vi "Graph Display.vi"(10 "telem notifier":refnum<notifier>) -> ()   [LabVIEW 2015]
uses:
  Telemetry Packet Type.ctl
  Thermocouple Data.ctl
  Transducer Calibration Display.ctl
  Sensor Enum.ctl
  Sensor Data Global Action.ctl
panel:
  out "Timestamp":u32
  out "Air Pressure":dbl(graph)
  out "Compressor Temperature":dbl(graph)
  out "Article Temperature":dbl(graph)
  out "Accumulator Pressures":cluster{"FPD-2":dbl, "OPD-2":dbl}(graph)
  out "Chamber Pressure":cluster{"PC-2":dbl, "PC-1":dbl}(graph)
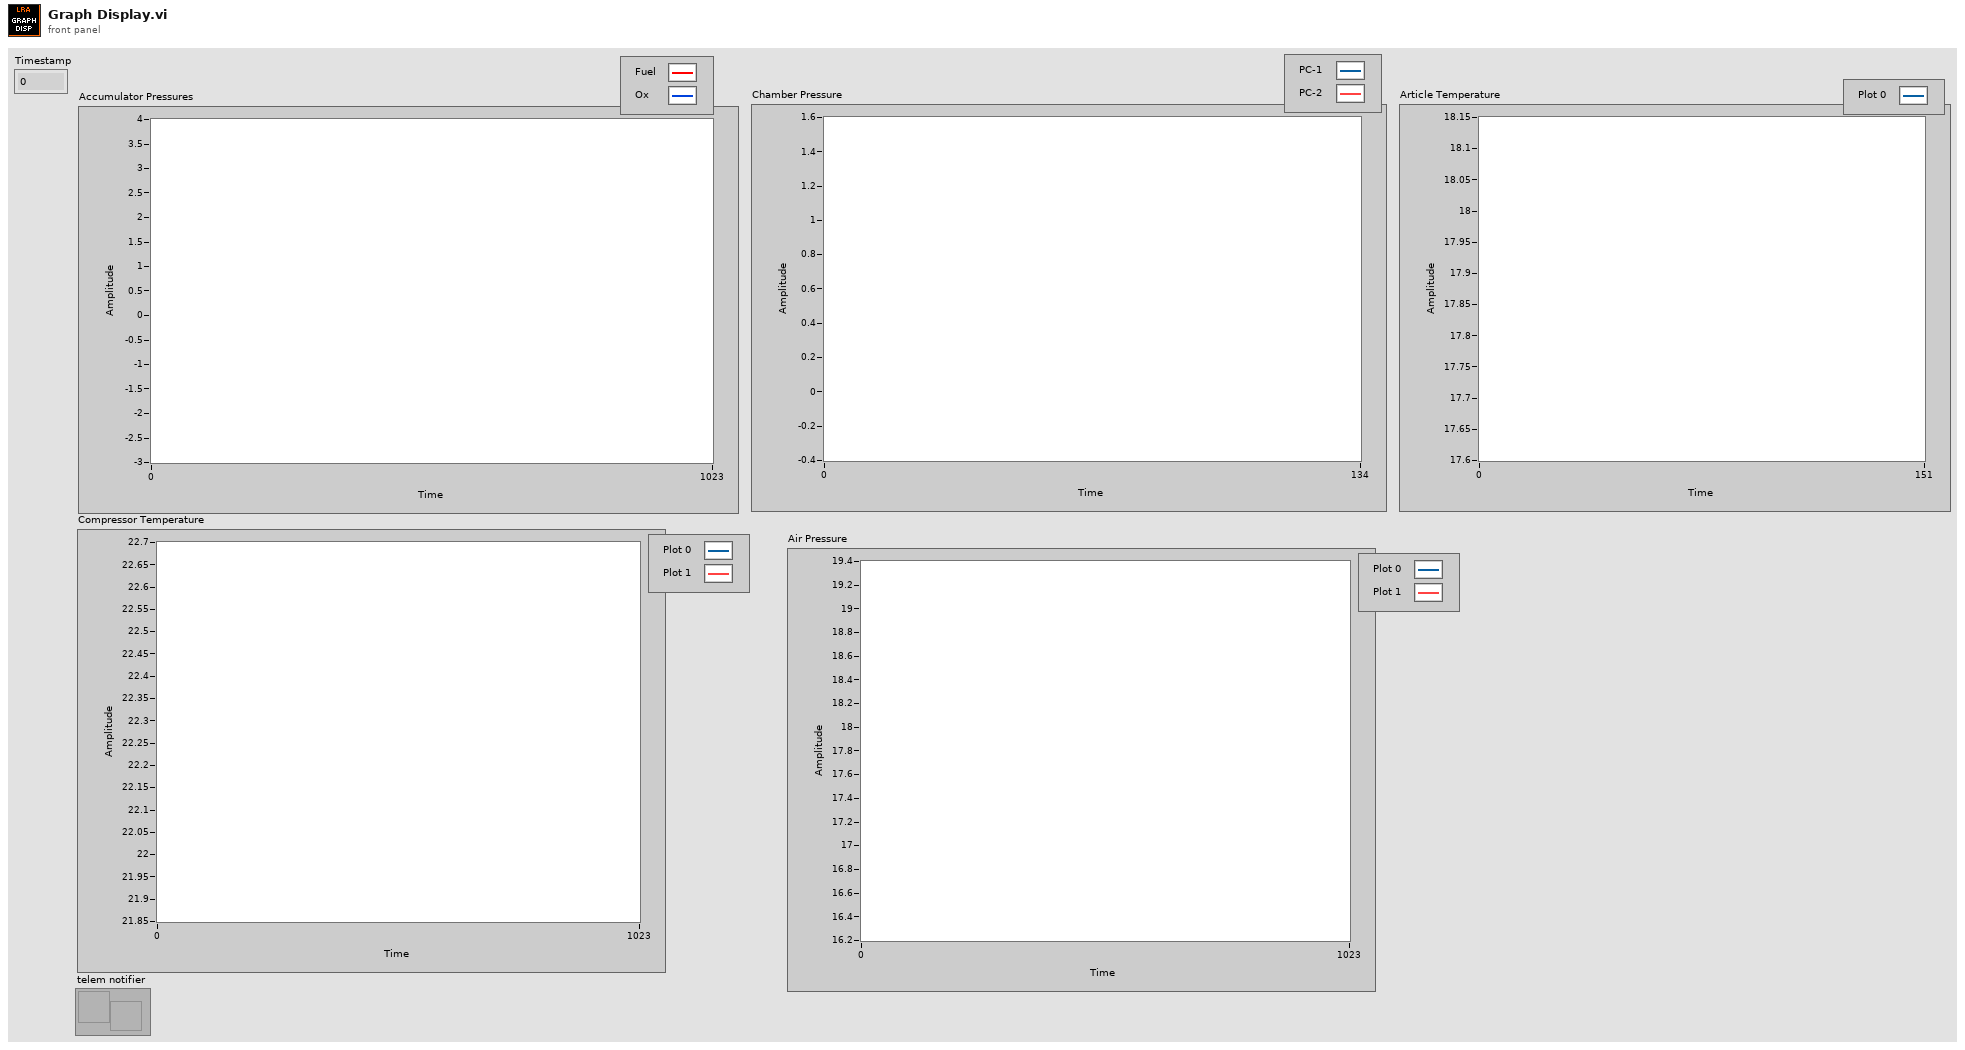
[diagram p1: front panel]
types:
  T1 = typedef "Sensor Enum.ctl" = enum16{"FPD-1", "FPD-2", "FPD-3", "OPD-1", "OPD-2", "OPD-3", "AP-1", "PC-1", "PC-2", "VBAT", "VCOMP", "ICOMP", "TC-1", "TC-COMP"}
  T2 = typedef "Sensor Data Global Action.ctl" = enum16{"Get Data", "Decode & Store Data"}
  T3 = typedef "Telemetry Packet Type.ctl" = cluster{"Timestamp\n":u32, "Transducer Value":u16[], "Main Loop Rate":u32, "Solenoid State":bool[], "Output Enabled":bool, "Solenoids Powered":bool, "TC Data":T4[], "TD Rate":u32, "TD Execution Time":u32, "TC Rate":u32, "TC Execution Time":u32, "Decoded Sensor Data":T5[], "Watchdog Expired?":bool}
  T4 = typedef "Thermocouple Data.ctl" = cluster{"TC Temp":dbl, "Internal Temp":dbl, "Fault":bool, "Short to VCC":bool, "Short to GND":bool, "Open Circuit":bool}
  T5 = typedef "Transducer Calibration Display.ctl" = cluster{"Value":dbl, "Raw":dbl, "Scaled":dbl, "Sensor Name":T1, "Port":u32}
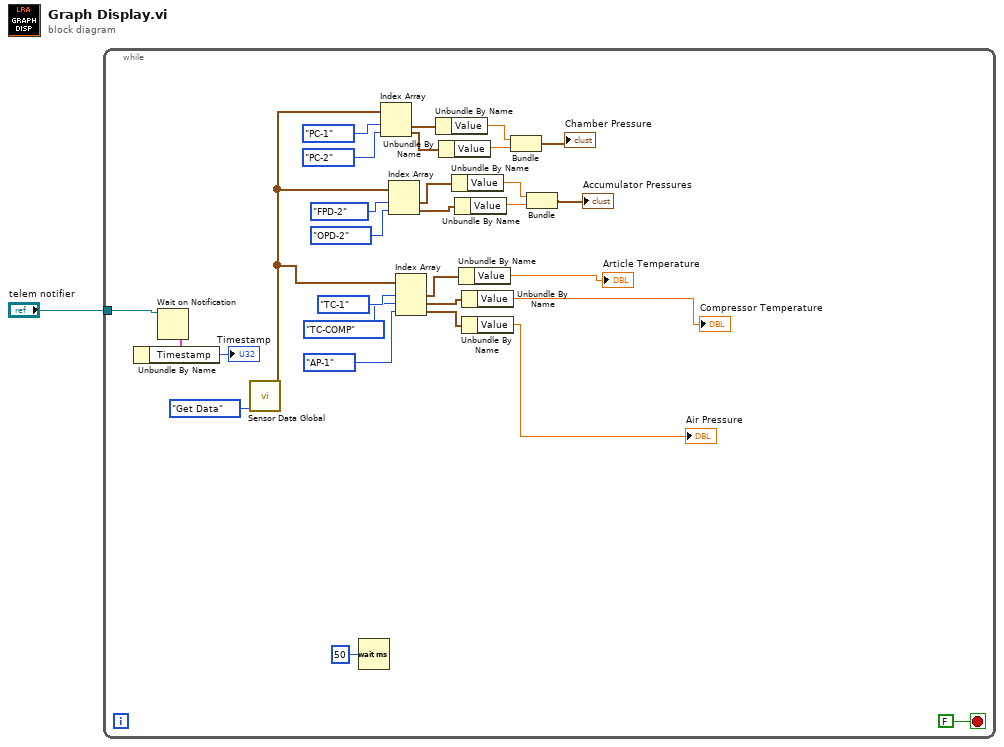
[diagram p0: block diagram]
diagram:
  n1 = while {
    tunnel: "telem notifier" -> [w30]
    stop <- FALSE stop-if-true
    n2 = Wait on Notification(notifier=w30) -> (notification=w29:T3)  [unwired: 3 in, 3 out]
    n3 = Unbundle By Name(w29) -> ("Timestamp"=→"Timestamp":u32)
    n4 = call "Sensor Data Global.vi"("Command"=Sensor_Data_Global_Action."Get Data") -> ("Sensor Data"=w10:T5[])  [unwired: 10 in]
    n5 = Wait (ms)(milliseconds to wait=u32 50) -> ()  [unwired: 1 out]
    n6 = Index Array(array=w10, index #1=Sensor_Enum."PC-1" ("Sensor Name"), index #2=Sensor_Enum."PC-2" ("Sensor Name")) -> (element #1=w25:T5, element #2=w24:T5)
    n7 = Index Array(array=w10, index #1=Sensor_Enum."FPD-2" ("Sensor Name"), index #2=Sensor_Enum."OPD-2" ("Sensor Name")) -> (element #1=w16:T5, element #2=w15:T5)
    n8 = Index Array(array=w10, index #1=Sensor_Enum."TC-1" ("Sensor Name"), index #2=Sensor_Enum."TC-COMP" ("Sensor Name"), index #3=Sensor_Enum."AP-1" ("Sensor Name")) -> (element #1=w9:T5, element #2=w13:T5, element #3=w5:T5)
    n9 = Unbundle By Name(w25) -> ("Value"=w23:dbl)
    n10 = Unbundle By Name(w24) -> ("Value"=w22:dbl)
    n11 = Unbundle By Name(w16) -> ("Value"=w17:dbl)
    n12 = Unbundle By Name(w15) -> ("Value"=w18:dbl)
    n13 = Unbundle By Name(w9) -> ("Value"=→"Article Temperature":dbl)
    n14 = Unbundle By Name(w13) -> ("Value"=→"Compressor Temperature":dbl)
    n15 = Unbundle By Name(w5) -> ("Value"=→"Air Pressure":dbl)
    n16 = Bundle("Value"=w23, "Value"=w22) -> (→"Chamber Pressure":cluster{"Value":dbl, "Value":dbl})  [unwired: 1 in]
    n17 = Bundle("Value"=w17, "Value"=w18) -> (→"Accumulator Pressures":cluster{"Value":dbl, "Value":dbl})  [unwired: 1 in]
  }
